vi "Core Action.vi"(8 "error in (no error)":errorcluster, 10 "SECS-II Class":refnum<class "SECS-II Class.lvclass">, 11 "08-Host Requsts Event Report in":refnum<class "08-Host Requsts Event Report.lvclass">) -> (0 "error out":errorcluster, 2 "SECS-II Class Out":refnum<class "SECS-II Class.lvclass">, 3 "08-Host Requsts Event Report out":refnum<class "08-Host Requsts Event Report.lvclass">)   [LabVIEW 2020, in "SECS Scenarios.lvlib" / "08-Host Requsts Event Report.lvclass"]
uses:
  08-Host Requsts Event Report.lvclass
  D:/Dropbox/SECS/SECS_GEM v1.1.0/Com/SECS Scenarios/Scenarios Class/Scenarios Class.lvclass
  SECS Communication/SECS-II Class/SECS-II Class.lvclass
  SECS Communication/S6 Message Class/S6 Message Class.lvclass
  D:/Dropbox/SECS/SECS_GEM v1.1.0/Com/SECS Communication/SECS-II Class/SECS-II Class.lvclass
  Scenarios Class/Reply State.ctl
  Scenarios Class/Scenarios Class.lvclass/Scenarios Class.ctl
  Scenarios Class/Write Reply State.vi
  Scenarios Class/Read HSMS Class.vi
  SECS Communication/HSMS Class/HSMS Class.lvclass
  Scenarios Class/Scenarios Class.lvclass
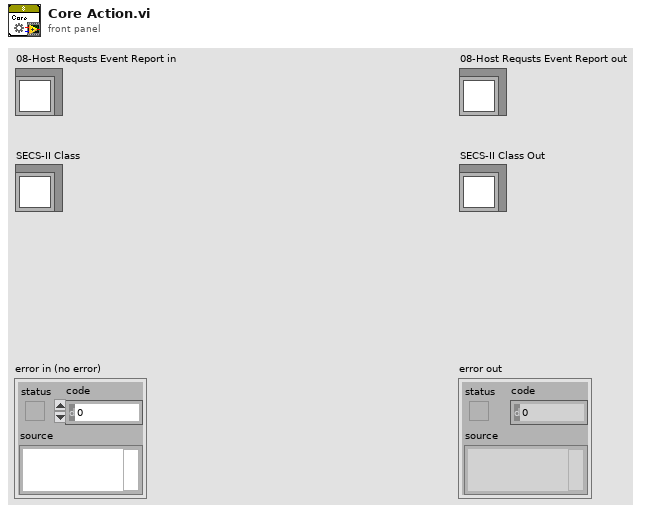
[diagram p1: front panel]
types:
  T1 = typedef "SECS Communication.lvlib/S6 Message Class.lvclass/S6F16.ctl" = cluster{"DATAID":u32, "CEID":u32, "Report Data":cluster{"RPTID":u32, "Value":cluster{"Format Code":T2, "Value":variant}[]}[]}
  T2 = typedef "SECS Communication.lvlib/SECS-II Class.lvclass/Format Code.ctl" = enum16{"L", "A", "B", "Boolean", "J", "I1", "I2", "I4", "I8", "U1", "U2", "U4", "U8", "F4", "F8", "Char"}
  T3 = typedef "SECS Scenarios.lvlib/Scenarios Class.lvclass/Reply State.ctl" = enum16{"OK", "Illegal Data", "Unknown Stream", "Unknown Function", "Off-Line", "T3 Timeout", "Inner-Timeout"}
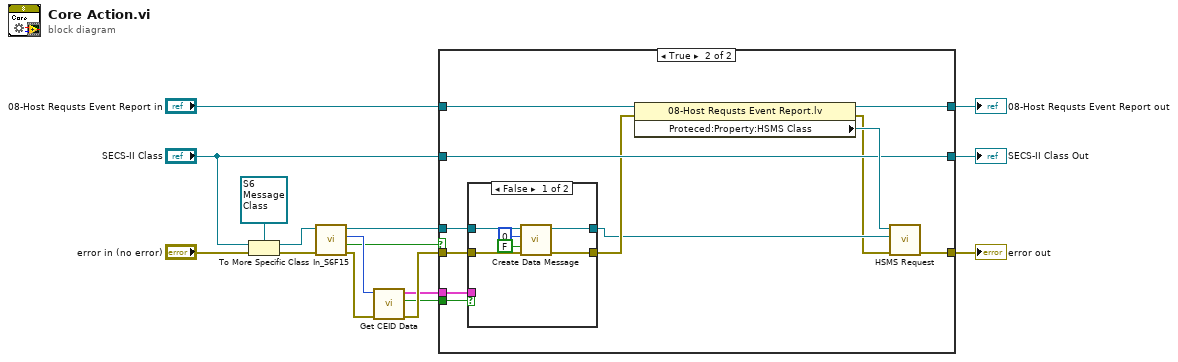
[diagram p0: block diagram]
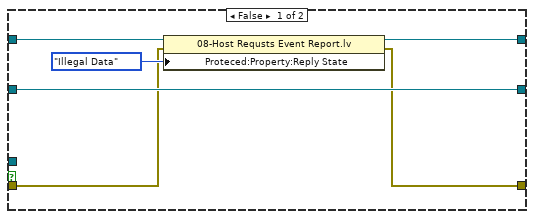
[diagram p2: hidden frame]
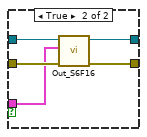
[diagram p3: hidden frame]
diagram:
  n1 = To More Specific Class(target class=refnum<class "S6 Message Class.lvclass"> refnum ("SECS Communication.lvlib:S6 Message Class.lvclass"), reference="SECS-II Class", error in="error in (no error)") -> (specific class reference=w15:refnum<class "S6 Message Class.lvclass">, error out=w16:errorcluster)
  n2 = call "In_S6F15.vi"("error in (no error)"=w16, "S6 Message Class in"=w15) -> ("error out"=w6:errorcluster, "OK?"=w1:bool, "CEID"=w5:u32, "S6 Message Class out"=w14:refnum<class "S6 Message Class.lvclass">)  [unwired: 6 in]
  n3 = call "Get CEID Data.vi"("error in (no error)"=w6, "CEID"=w5) -> ("error out"=w4:errorcluster, "OK?"=w3:bool, "S6F16"=w2:T1)  [unwired: 7 in]
  n4 = case shown="True" w1 {
    tunnel: "08-Host Requsts Event Report in" -> [w21 w34]
    tunnel: [w20 w33] -> w13
    tunnel: [w19 w32] -> w12
    tunnel: w14 -> [_ w27]
    tunnel: "SECS-II Class" -> [w22 w30]
    tunnel: [w22 w30] -> w7
    tunnel: w4 -> [w17 w25]
    tunnel: w3 -> [_ w29]
    tunnel: w2 -> [_ w28]
    frame False {
      n5 = property class="08-Host Requsts Event Report.lv"(reference=w21, error in=w17, "Proteced:Property:Reply State"=Reply_State."Illegal Data" ("Reply State")) -> (reference out=w20:refnum<class "08-Host Requsts Event Report.lvclass">, error out=w19:errorcluster)
    }
    frame True {
      n6 = case shown="False" w29 {
        tunnel: w28 -> [_ w43]
        tunnel: w27 -> [w40 w45]
        tunnel: [w39 w42] -> w24
        tunnel: [w38 w41] -> w26
        tunnel: w25 -> [w37 w44]
        frame False {
          n7 = call "Create Data Message.vi"("error in (no error)"=w37, "W-Bit"=FALSE, "Function"=u8 0, "SECS-II Class in"=w40) -> ("error out"=w38:errorcluster, "SECS-II Class out"=w39:refnum<class "S6 Message Class.lvclass">)  [unwired: 6 in]
        }
        frame True {
          n8 = call "Out_S6F16.vi"("error in (no error)"=w44, "S6F16"=w43, "S6 Message Class in"=w45) -> ("error out"=w41:errorcluster, "S6 Message Class out"=w42:refnum<class "S6 Message Class.lvclass">)  [unwired: 7 in]
        }
      }
      n9 = property class="08-Host Requsts Event Report.lv"(reference=w34, error in=w26) -> (reference out=w33:refnum<class "08-Host Requsts Event Report.lvclass">, error out=w23:errorcluster, "Proteced:Property:HSMS Class"=w31:refnum<class "HSMS Class.lvclass">)
      n10 = call "HSMS Request.vi"("error in (no error)"=w23, "SECS-II Class In"=w24, "HSMS Class in"=w31) -> ("error out"=w32:errorcluster)  [unwired: 7 in, 1 out]
    }
  }
  "error out" <- w12
  "08-Host Requsts Event Report out" <- w13
  "SECS-II Class Out" <- w7
